vi "Exit.vi"(8 "error in (no error)":errorcluster, 11 "Old State":refnum<class "Idle.lvclass">) -> (0 "error out":errorcluster, 3 "New State":refnum<class "Idle.lvclass">)   [LabVIEW 2024, in "Chef State.lvlib" / "Idle.lvclass"]
doc: "This is an abstract method. Override this method to define the behavior when you leave the state."
uses:
  Idle.lvclass
  C:/Program Files/National Instruments/LabVIEW 2024/vi.lib/ActorFramework/Actor/Actor.lvclass
  <vilib>/ActorFramework/Actor/Actor.lvclass/Actor.ctl
  Chef UI Logic/Chef UI Logic Messages/Update Log Msg/Update Log Msg.lvclass/Update Log Msg.ctl
  <vilib>/ActorFramework/Message Enqueuer/Message Enqueuer.lvclass/Message Enqueuer.ctl
  <vilib>/ActorFramework/Message Enqueuer/Enqueue.vi
  Chef UI Logic/Chef UI Logic Messages/Update Log Msg/Update Log Msg.lvclass
  C:/Program Files/National Instruments/LabVIEW 2024/vi.lib/ActorFramework/Message/Message.lvclass
  <vilib>/ActorFramework/Message Priority Queue/Priority Enqueue.vi
  Chef State/Chef State.lvclass
  Idle.lvclass/Idle.ctl
  <vilib>/ActorFramework/Actor/Actor.lvclass
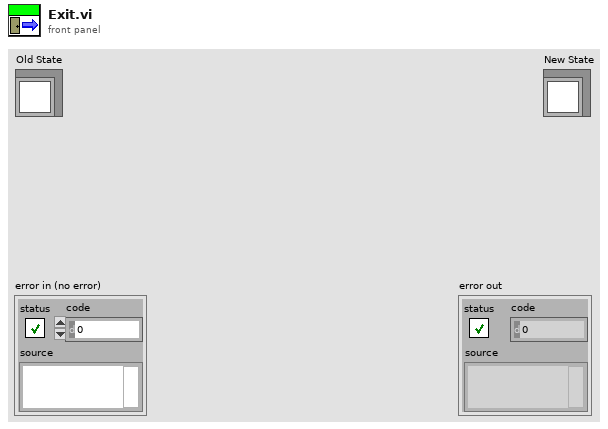
[diagram p1: front panel]
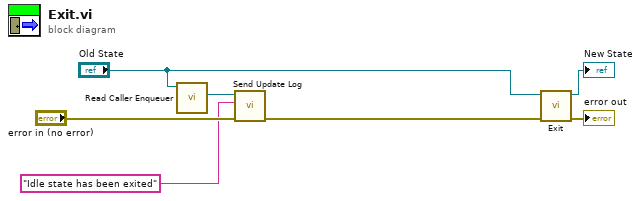
[diagram p0: block diagram]
diagram:
  n1 = call <vilib>:"Read Caller Enqueuer.vi"("Actor"="Old State") -> ("Caller Enqueuer"=w4:refnum<class "Message Enqueuer.lvclass">)  [unwired: 10 in]
  n2 = call "Send Update Log.vi"("error in (no error)"="error in (no error)", "Log"="Idle state has been exited", "Message Enqueuer"=w4) -> ("error out"=w2:errorcluster)  [unwired: 7 in, 1 out]
  n3 = call-parent "Exit.vi"("error in (no error)"=w2, "Old State"="Old State") -> ("error out"=→"error out":errorcluster, "New State"=→"New State":refnum<class "Idle.lvclass">)  [unwired: 8 in]
